vi "CIB Cal UI.vi"(11 "Calling VI Ref":refnum<vi>) -> ()   [LabVIEW 2013]
uses:
  Type Defs/Cal Point Type Def.ctl
  <vilib>/Utility/miscctls.llb/LVRowAndColumnTypeDef.ctl
panel:
  in  "debug":bool=TRUE
  in  "Load Indicator Tab":enum32{"Page 1"}(tab)
  in  "Header Tab":enum32{"Page 1", "Page 2"}(tab)
  in  "Header OK":bool
  in  "Header Cancel":bool
  in  "Header Comments":string[][](table)=[["PRODUCT 5V. IS REFERENCE ONLY."], ["1"], ["2"]]
  in  "Cal Standards Table":string[][](table)=[["FLUKE MULTIMETER", "3539"], ["FLUKE CALIBRATOR", "7955"], ["", ""], ["", ""], ["", ""]]
  in  "Sys Cal Table":string[][](table)=[["CIB BD.", "DSS 9372-1"], ["D/A BD.", "DSS 9372-2"], ["", ""], ["", ""], ["", ""]]
  in  "Header Table 1":string[][](table)=[["9372blah"], ["DELPHI"], ["TL1181E"], ["EU2C397"], ["CIB/ D/A BD."], ["5 VOLTS"], ["NEW"], ["9087"]]
  in  "Header Table 2":string[][](table)=[["39687"], ["12"], ["40052"], ["MDC"], ["24"], ["48"], ["JUM  /   DR"]]
  in  "Main Tab":enum32{"Page 1", "Page 2"}(tab)
  in  "Address":string
  in  "Send 485 Cmd":bool
  in  "485 Command":string(combo)="p_on"
  in  "View Spreadsheet":bool
  in  "Confirm Point":bool
  in  "Header":bool
  in  "Cal Point":T1
  out "CIB SN":string caption="CIB Serial Number"
  out "Dev Table 1":string[][](table)
  in  "Actual Table 1":string[][](table)=[[""], [""], [""], [""], [""], [""], [""], [""], [""]]
  out "Actual Table 2":string[][](table)
  out "Dev Table 2":string[][](table)
  in  "Read CIB":bool
  # "System Calibration Components"
  # "Calibration Standards Used"
  # "1) Enter Header Information"
  # "Send 485 Command"
  # "2) Select Cal Point"
  # "3) Collect Data"
  # "4)  Confirm/Review"
  # "*Excel must be closed to return control to this app."
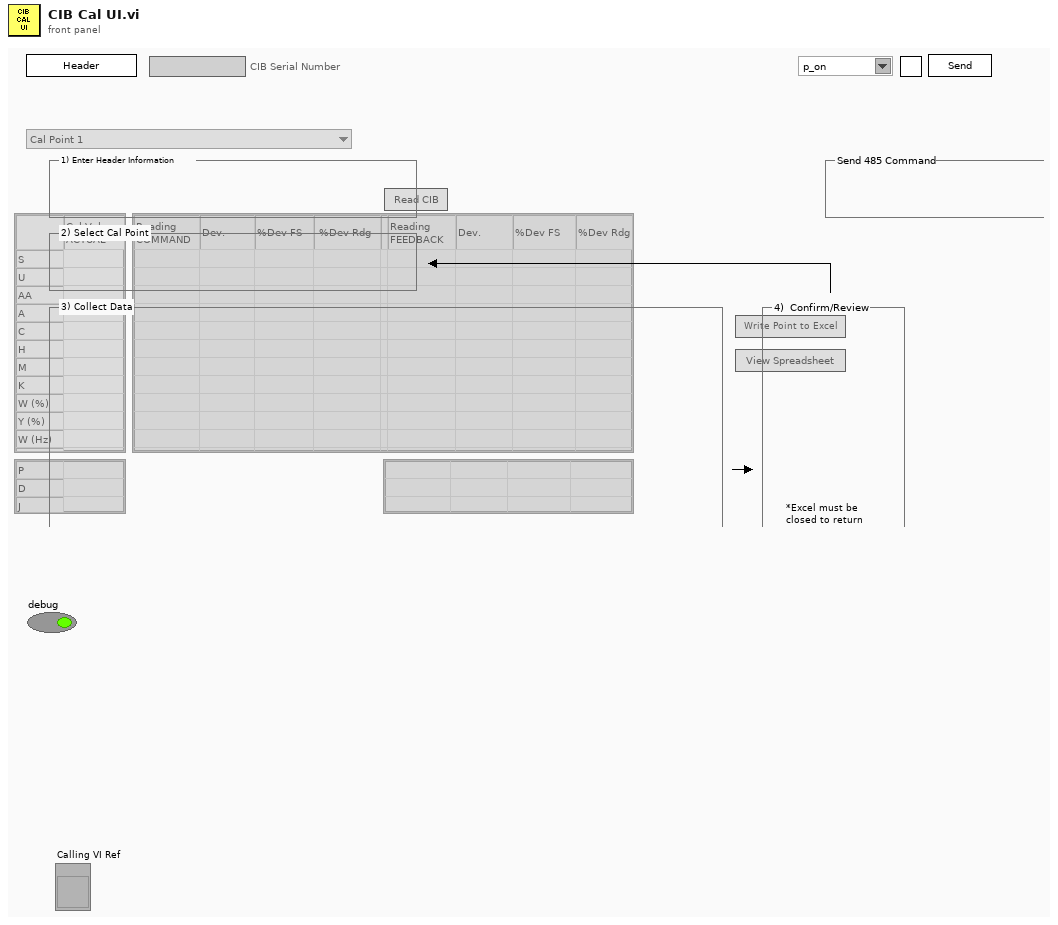
[diagram p1: front panel]
types:
  T1 = typedef "Cal Point Type Def.ctl" = enum16{"Cal Point 1", "Cal Point 2", "Cal Point 3", "Cal Point 4", "Cal Point 5", "Cal Point 6", "Cal Point 7"}
  T2 = cluster{"Error":errorcluster, "Cal Files Path":path, "Base Path":path, "Calling VI Ref":refnum<vi>, "Cal Template Path":path, "Current Cal Path":path, "Cal Point":T1, "Actual Table 1":string[][], "Actual Table 2":string[][], "Dev Table 1":string[][], "Dev Table 2":string[][], "Dev Table 1 Ref":refnum<vi>, "Dev Table 2 Ref":refnum<vi>, "COM Ref":refnum<visa-resource-name>, "COM Found":bool, "debug":bool, "Read CIB":bool}
  T3 = enum8{"Enabled", "Disabled", "Disabled and Grayed Out"}
  T4 = typedef "LVRowAndColumnTypeDef.ctl" = cluster{"Row":i32, "Column":i32}
  T5 = enum32{"Bad", "Idle", "Run top level", "Running"}
  T6 = typedef "eventvkey.ctl" = enum16{"ASCII", "Enter", "Return", "Shift", "Ctrl", "Alt", "Cmd", "Opt", "Caps", "NumLock", "Clear", "Break", "Up", "Down", "Left", "Right", "Insert", "Delete", "Home", "End", "PageUp", "PageDown", "Escape", "Help", "Pause", "ScrollLock", "F1", "F2", "F3", "F4", "F5", "F6", "F7", "F8", "F9", "F10", "F11", "F12", "F13", "F14", "F15", "F16", "F17", "F18", "F19", "F20", "F21", "F22", "F23", "F24", "Play", "VolumeUp", "VolumeDown", "Mute", "Two Byte Char"}
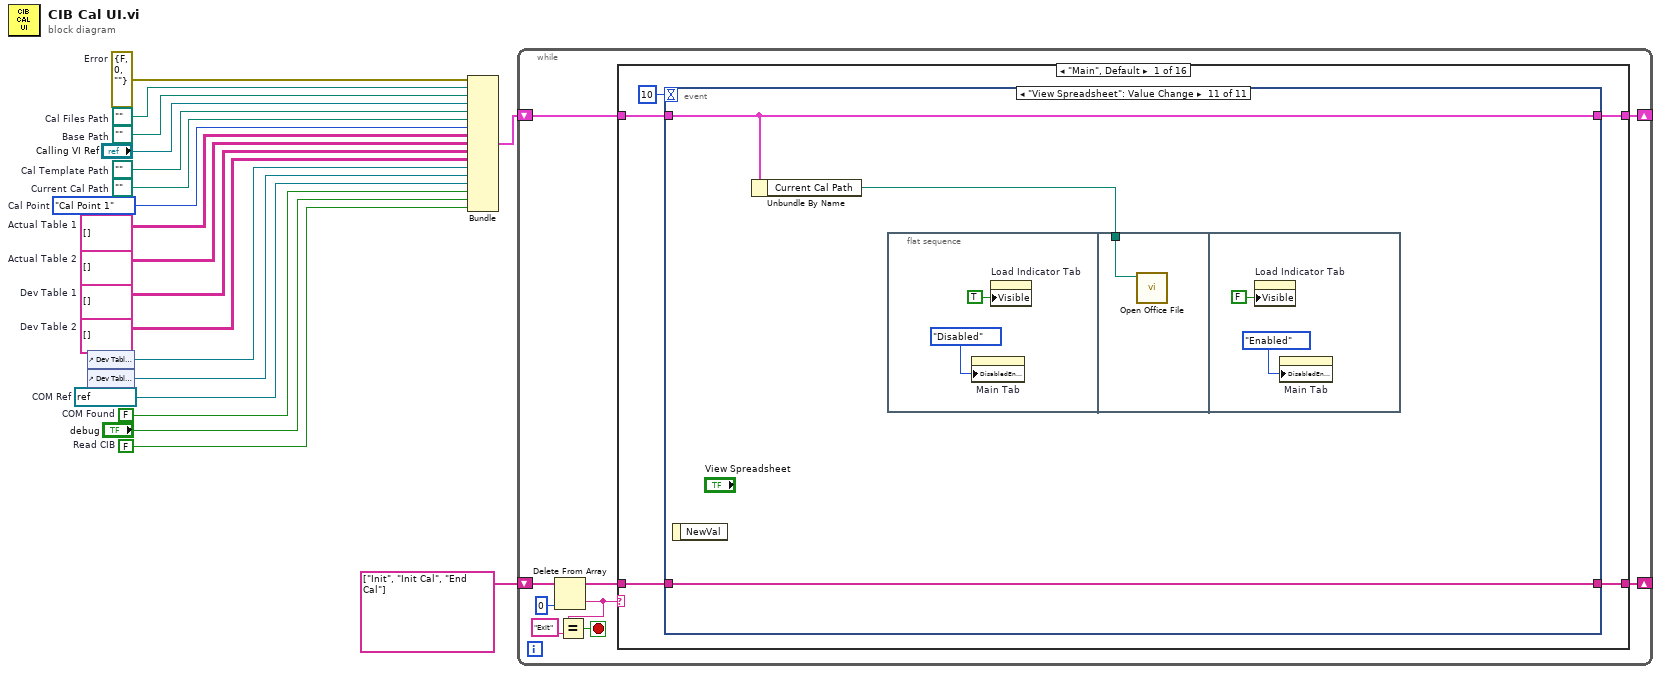
[diagram p0: block diagram]
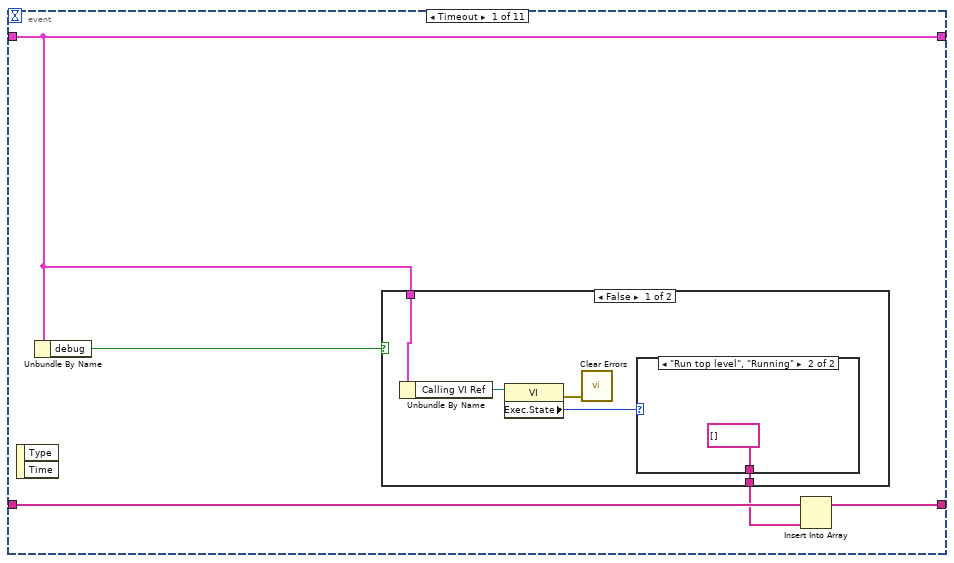
[diagram p2: hidden frame]
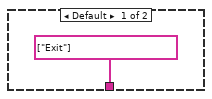
[diagram p3: hidden frame]
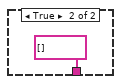
[diagram p4: hidden frame]
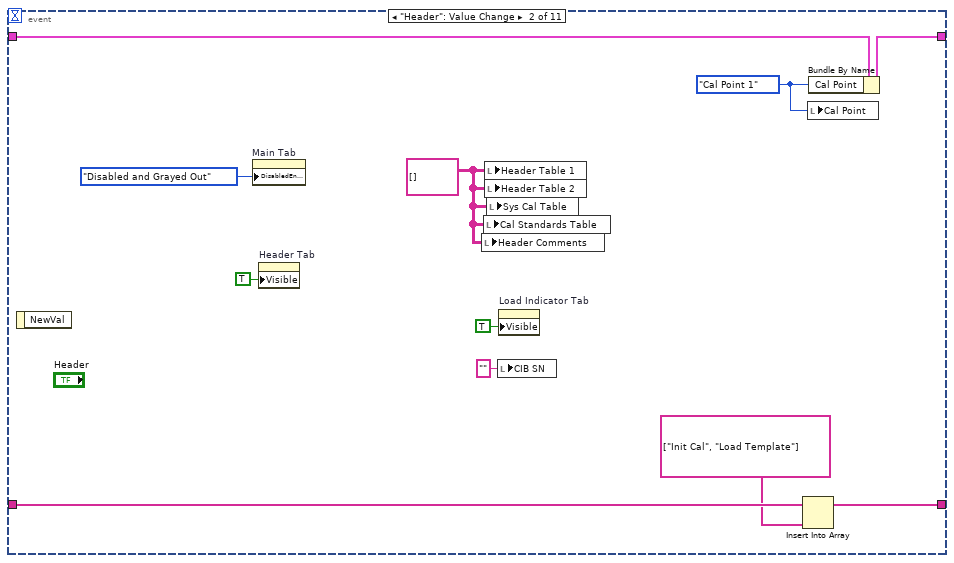
[diagram p5: hidden frame]
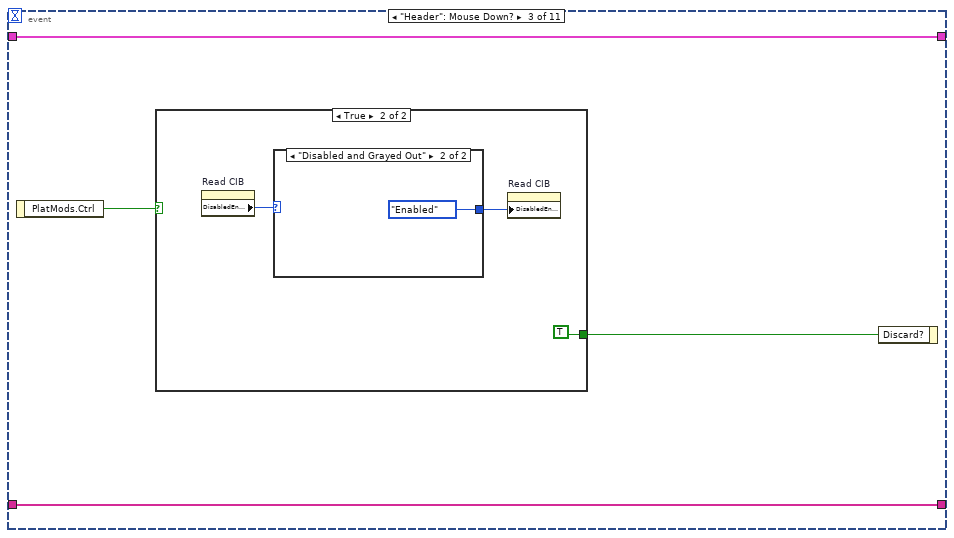
[diagram p6: hidden frame]
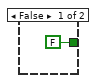
[diagram p7: hidden frame]
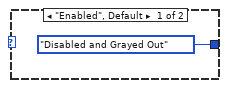
[diagram p8: hidden frame]
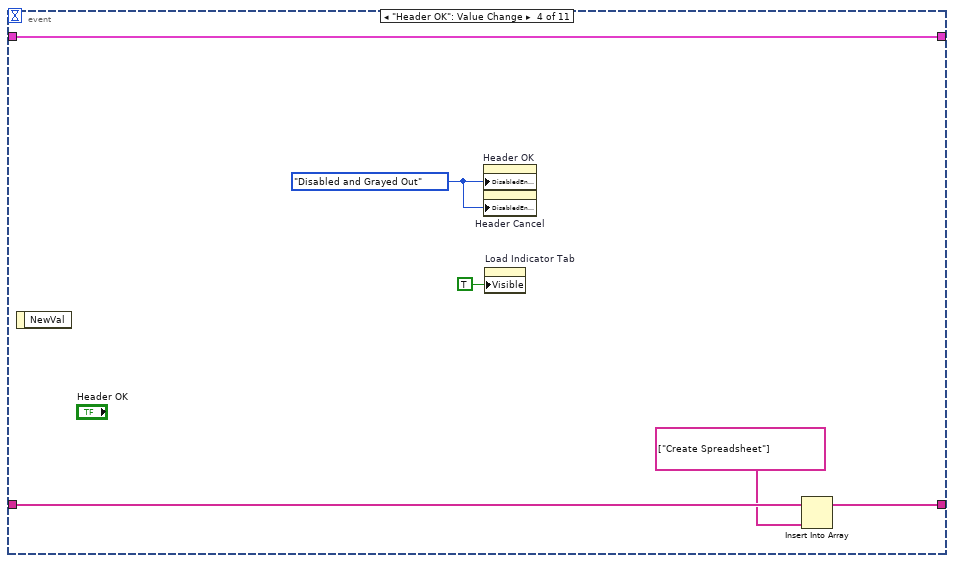
[diagram p9: hidden frame]
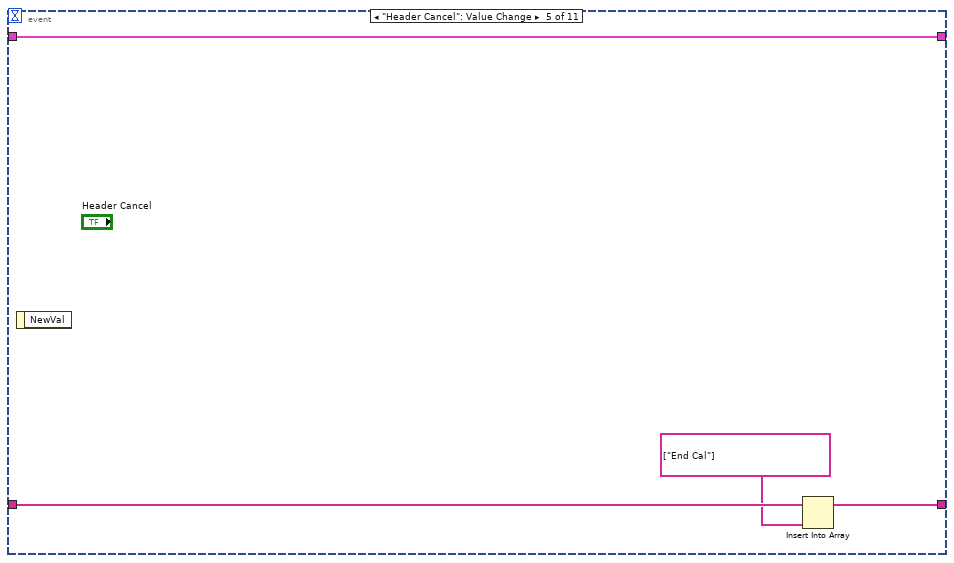
[diagram p10: hidden frame]
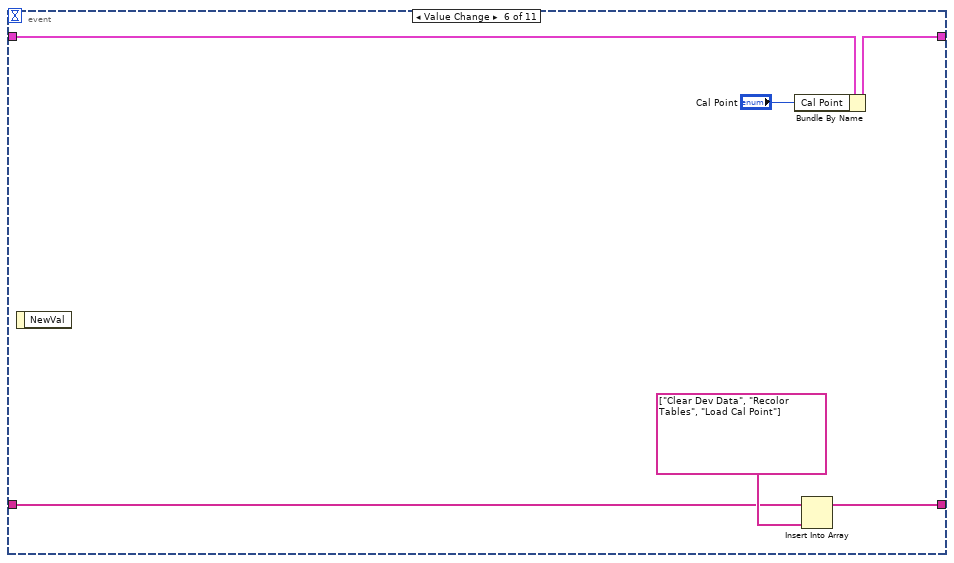
[diagram p11: hidden frame]
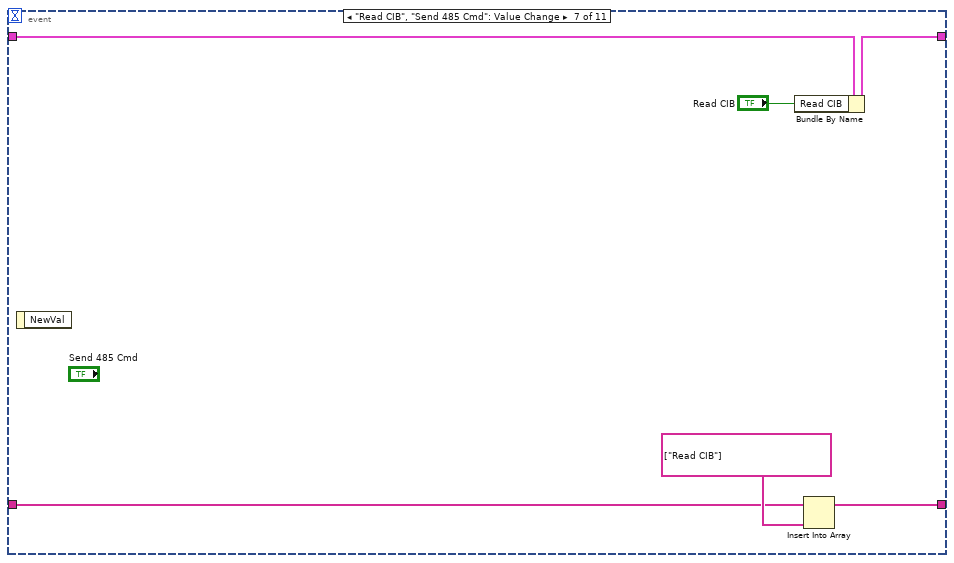
[diagram p12: hidden frame]
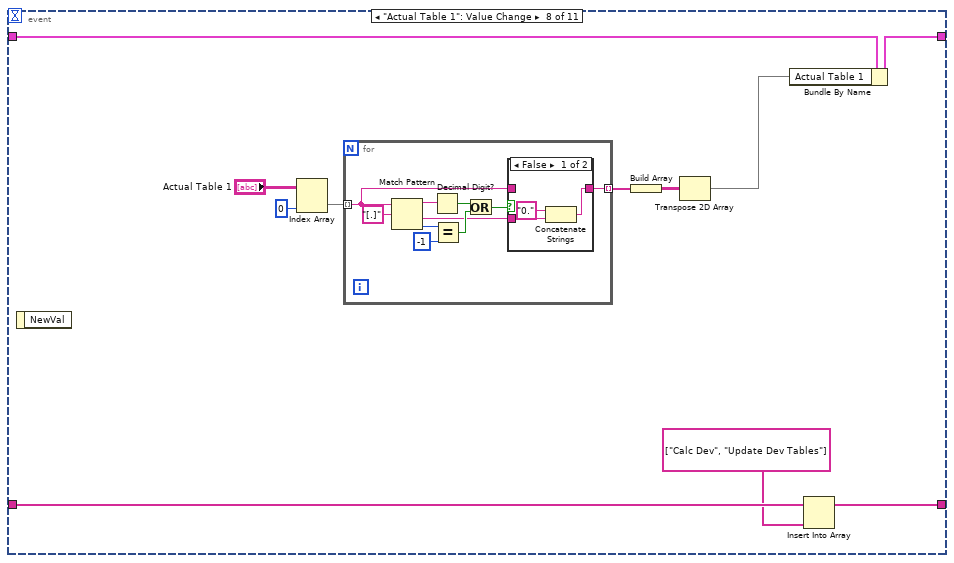
[diagram p13: hidden frame]
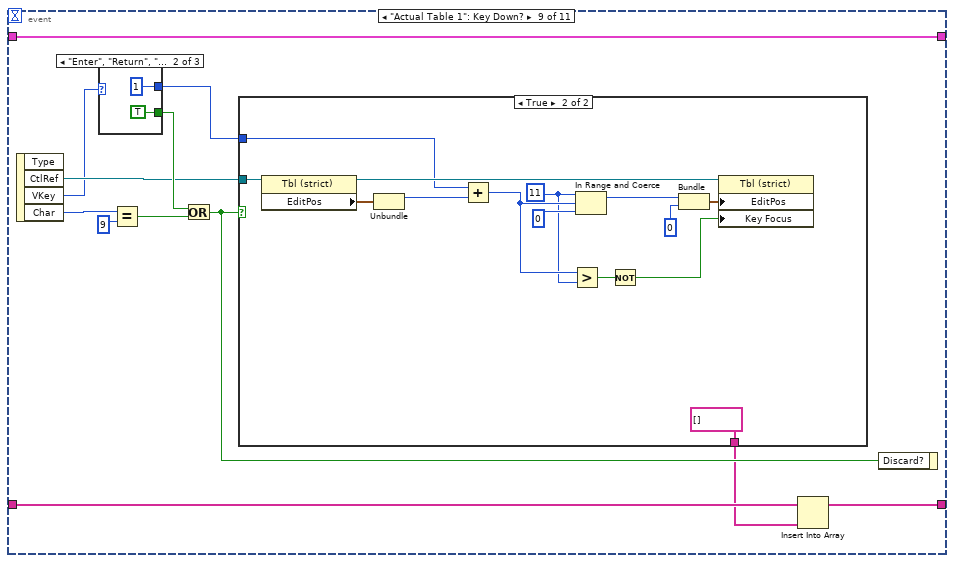
[diagram p15: hidden frame]
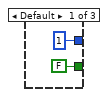
[diagram p16: hidden frame]
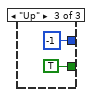
[diagram p17: hidden frame]
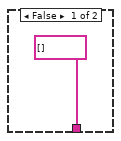
[diagram p18: hidden frame]
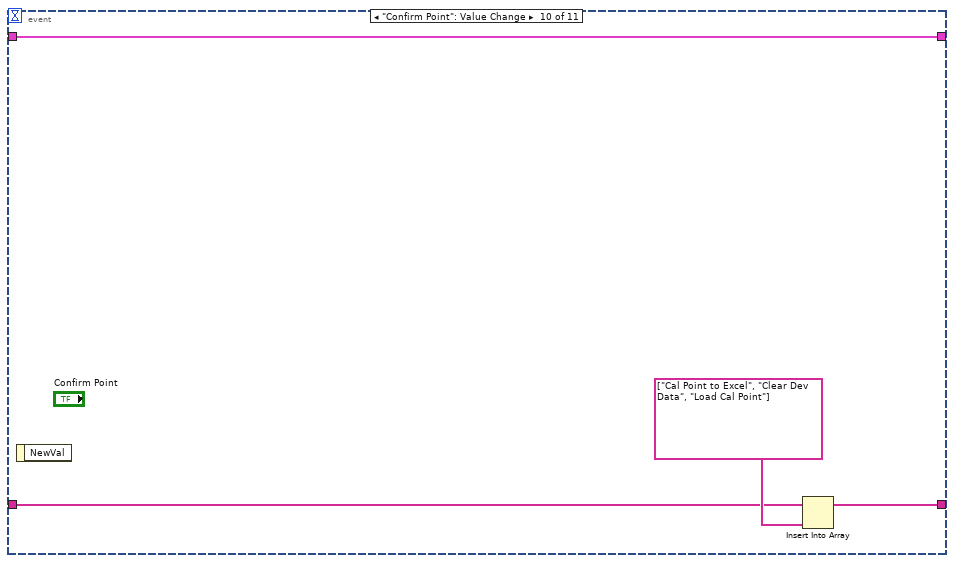
[diagram p19: hidden frame]
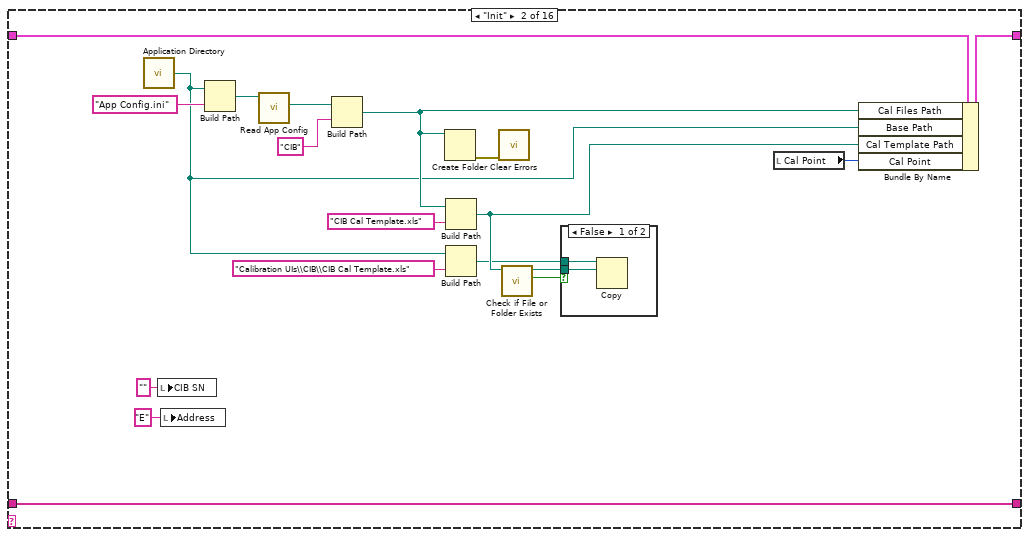
[diagram p20: hidden frame]
diagram:
  w1 = FALSE  # Read CIB
  w3 = FALSE  # COM Found
  w4 = refnum<visa-resource-name> "COM4"  # COM Ref
  w7 = string[][] []  # Dev Table 2
  w8 = string[][] []  # Dev Table 1
  w9 = string[][] []  # Actual Table 2
  w10 = string[][] []  # Actual Table 1
  w11 = Cal_Point_Type_Def."Cal Point 1"  # Cal Point
  w12 = path ""  # Current Cal Path
  w13 = path ""  # Cal Template Path
  w15 = path ""  # Base Path
  w17 = path ""  # Cal Files Path
  w16 = errorcluster {"status"=FALSE, "code"=0, "source"=""}  # Error
  n1 = control-ref of="Dev Table 1 Ref"() -> (w6:refnum<vi>)
  n2 = control-ref of="Dev Table 2 Ref"() -> (w5:refnum<vi>)
  n3 = Bundle("Error"=w16, "Cal Files Path"=w17, "Base Path"=w15, "Calling VI Ref"="Calling VI Ref", "Cal Template Path"=w13, "Current Cal Path"=w12, "Cal Point"=w11, "Actual Table 1"=w10, "Actual Table 2"=w9, "Dev Table 1"=w8, "Dev Table 2"=w7, "Dev Table 1 Ref"=w6, "Dev Table 2 Ref"=w5, "COM Ref"=w4, "COM Found"=w3, "debug"="debug", "Read CIB"=w1) -> (w18:T2)  [unwired: 1 in]
  n4 = while {
    shift-right: [w25] -> _
    shift-left: string[] ["Init", "Init Cal", "End Cal"] -> [w28]
    shift-right: [w21] -> _
    shift-left: w18 -> [w22]
    stop <- w27 stop-if-true
    n5 = Delete From Array(array=w28, index=0) -> (deleted portion=w24:string, array with subset deleted=w26:string[])  [unwired: 1 in]
    n6 = Equal?(x=w24, y="Exit" ("x")) -> (x = y?=w27:bool)
    n7 = case shown="\"Main\", Default" w24 {
      tunnel: [w31 w174 w181 w185 w194 w204 w238 w273 w309 w343 w363 w426 w455 w489 w502 w504] -> w25
      tunnel: w26 -> [w32 w174 w181 w184 w193 w203 w237 w272 w308 w342 w362 w425 w454 w489 w501 w504]
      tunnel: w22 -> [w30 w178 w182 w183 w192 w201 w229 w270 w307 w341 w366 w429 w450 w488 w493 w503]
      tunnel: [w29 w177 w182 w183 w191 w201 w228 w270 w306 w341 w365 w428 w449 w488 w493 w503] -> w21
      frame "Main", Default {
        n8 = event shown="[10] \"View Spreadsheet\": Value Change" {
          selector: _ -> [_ _ _ _ _ _ _ _ _ _ _]
          dyn-events: _ -> [_ _ _ _ _ _ _ _ _ _ _]
          timeout: 10 -> [_ _ _ _ _ _ _ _ _ _ _]
          tunnel: [w38 w57 w60 w72 w76 w79 w88 w100 w118 w150 w154] -> w31
          tunnel: w32 -> [w37 w56 w60 w71 w75 w78 w87 w99 w117 w149 w154]
          tunnel: [w35 w48 w61 w73 w77 w82 w85 w97 w115 w148 w153] -> w29
          tunnel: w30 -> [w35 w49 w61 w73 w77 w83 w86 w98 w115 w148 w153]
          event Timeout {
            n9 = event-data() -> ()  [unwired: 1 in, 2 out]
            n10 = Unbundle By Name(w35) -> ("debug"=w34:bool)
            n11 = case shown="False" w34 {
              tunnel: [w43 string[] []] -> w36
              tunnel: w35 -> [w40 _]
              frame False {
                n12 = Unbundle By Name(w40) -> ("Calling VI Ref"=w42:refnum<vi>)
                n13 = property class="VI"(reference=w42) -> (error out=w39:errorcluster, "Exec.State"=w41:T5)  [unwired: 1 in, 1 out]
                n14 = call <vilib>:"Clear Errors.vi"("error in (no error)"=w39) -> ()  [unwired: 6 in, 1 out]
                n15 = case shown="\"Run top level\", \"Running\"" w41 {
                  tunnel: [string[] ["Exit"] string[] []] -> w43
                  frame Default {
                  }
                  frame "Run top level", "Running" {
                  }
                }
              }
              frame True {
              }
            }
            n16 = Insert Into Array(array=w37, new element=w36) -> (w38:string[])  [unwired: 1 in]
          }
          event "Header": Value Change {
            w47 = Cal_Point_Type_Def."Cal Point 1" ("Cal Point")
            w53 = string[][] [] ("Header Table 1")
            n17 = event-data() -> ()  [unwired: 1 in, 1 out]
            n18 = property on="Main Tab" class="TabCtl (strict)"("DisabledEnum"=T3."Disabled and Grayed Out" ("Disabled")) -> ()  [unwired: 2 in, 2 out]
            n19 = property on="Header Tab" class="TabCtl (strict)"("Visible"=TRUE) -> ()  [unwired: 2 in, 2 out]
            n20 = local write "Header Comments"(w53) -> ()
            n21 = local write "Cal Standards Table"(w53) -> ()
            n22 = local write "Header Table 1"(w53) -> ()
            n23 = local write "Header Table 2"(w53) -> ()
            n24 = local write "Sys Cal Table"(w53) -> ()
            n25 = local write "CIB SN"("" ("CIB SN")) -> ()
            n26 = property on="Load Indicator Tab" class="TabCtl (strict)"("Visible"=TRUE) -> ()  [unwired: 2 in, 2 out]
            n27 = Insert Into Array(array=w56, new element=string[] ["Init Cal", "Load Template"]) -> (w57:string[])  [unwired: 1 in]
            n28 = local write "Cal Point"(w47) -> ()
            n29 = Bundle By Name(cluster=w49, "Cal Point"=w47) -> (w48:T2)
          }
          event "Header": Mouse Down? {
            n30 = event-data() -> ("PlatMods.Ctrl"=w59:bool)  [unwired: 1 in]
            n31 = case shown="True" w59 {
              tunnel: [FALSE TRUE] -> w58
              frame False {
              }
              frame True {
                n32 = property on="Read CIB" class="Bool"() -> ("DisabledEnum"=w65:T3)  [unwired: 2 in, 2 out]
                n33 = case shown="\"Disabled and Grayed Out\"" w65 {
                  tunnel: [T3."Disabled and Grayed Out" ("Disabled") T3."Enabled" ("Disabled")] -> w64
                  frame "Enabled", Default {
                  }
                  frame "Disabled and Grayed Out" {
                  }
                }
                n34 = property on="Read CIB" class="Bool"("DisabledEnum"=w64) -> ()  [unwired: 2 in, 2 out]
              }
            }
            n35 = event-data("Discard?"=w58) -> ()  [unwired: 1 in, 1 out]
          }
          event "Header OK": Value Change {
            w69 = T3."Disabled and Grayed Out" ("Disabled")
            n36 = event-data() -> ()  [unwired: 1 in, 1 out]
            n37 = property on="Header OK" class="Bool"("DisabledEnum"=w69) -> ()  [unwired: 2 in, 2 out]
            n38 = property on="Header Cancel" class="Bool"("DisabledEnum"=w69) -> ()  [unwired: 2 in, 2 out]
            n39 = property on="Load Indicator Tab" class="TabCtl (strict)"("Visible"=TRUE) -> ()  [unwired: 2 in, 2 out]
            n40 = Insert Into Array(array=w71, new element=string[] ["Create Spreadsheet"]) -> (w72:string[])  [unwired: 1 in]
          }
          event "Header Cancel": Value Change {
            n41 = event-data() -> ()  [unwired: 1 in, 1 out]
            n42 = Insert Into Array(array=w75, new element=string[] ["End Cal"]) -> (w76:string[])  [unwired: 1 in]
          }
          event Value Change {
            n43 = event-data() -> ()  [unwired: 1 in, 1 out]
            n44 = Bundle By Name(cluster=w83, "Cal Point"="Cal Point") -> (w82:T2)
            n45 = Insert Into Array(array=w78, new element=string[] ["Clear Dev Data", "Recolor Tables", "Load Cal Point"]) -> (w79:string[])  [unwired: 1 in]
          }
          event "Read CIB", "Send 485 Cmd": Value Change {
            n46 = event-data() -> ()  [unwired: 1 in, 1 out]
            n47 = Bundle By Name(cluster=w86, "Read CIB"="Read CIB") -> (w85:T2)
            n48 = Insert Into Array(array=w87, new element=string[] ["Read CIB"]) -> (w88:string[])  [unwired: 1 in]
          }
          event "Actual Table 1": Value Change {
            n49 = event-data() -> ()  [unwired: 1 in, 1 out]
            n50 = Index Array(array="Actual Table 1", index (col)=0 ("disabled index (col)")) -> (element=w94:string[])  [unwired: 1 in]
            n51 = for {
              tunnel: w94 -> [w103] mode=indexing
              tunnel: [w101] -> w93 mode=indexing
              n52 = Match Pattern(string=w103, regular expression="[.]") -> (before substring=w109:string, after substring=w102:string, offset past match=w107:i32)  [unwired: 1 in, 1 out]
              n53 = Decimal Digit?(1:w109) -> (0:w108:bool)
              n54 = Equal?(x=w107, y=-1) -> (x = y?=w105:bool)
              n55 = Or(x=w108, y=w105) -> (x .or. y?=w104:bool)
              n56 = case shown="False" w104 {
                tunnel: [w111 w114] -> w101
                tunnel: w103 -> [_ w114]
                tunnel: w102 -> [w113 _]
                frame False {
                  n57 = Concatenate Strings("0." ("string"), w113) -> (w111:string)
                }
                frame True {
                }
              }
            }
            n58 = Build Array(w93) -> (w92:string[][])
            n59 = Transpose 2D Array(2D array=w92) -> (transposed array=w90:string[][])
            n60 = Bundle By Name(cluster=w98, "Actual Table 1"=w90) -> (w97:T2)
            n61 = Insert Into Array(array=w99, new element=string[] ["Calc Dev", "Update Dev Tables"]) -> (w100:string[])  [unwired: 1 in]
          }
          event "Actual Table 1": Key Down? {
            n62 = event-data() -> ("CtlRef"=w122:refnum<vi>, "VKey"=w120:T6, "Char"=w121:i16)  [unwired: 1 in, 1 out]
            n63 = case shown="\"Enter\", \"Return\", \"Down\"" w120 {
              tunnel: [1 ("Column") 1 ("Column") -1 ("Column")] -> w125
              tunnel: [FALSE TRUE TRUE] -> w126
              frame Default {
              }
              frame "Enter", "Return", "Down" {
              }
              frame "Up" {
              }
            }
            n64 = Equal?(x=w121, y=i16 9) -> (x = y?=w123:bool)
            n65 = Or(x=w126, y=w123) -> (x .or. y?=w119:bool)
            n66 = case shown="True" w119 {
              tunnel: w122 -> [_ w147]
              tunnel: w125 -> [_ w142]
              tunnel: [string[] [] string[] []] -> w116
              frame False {
              }
              frame True {
                w136 = 11 ("y")
                n67 = property class="Tbl (strict)"(reference=w147) -> (reference out=w144:refnum<vi>, "EditPos"=w146:T4)  [unwired: 1 in, 1 out]
                n68 = Unbundle(w146) -> ("Row"=w141:i32)  [unwired: 1 out]
                n69 = Add(x=w142, y=w141) -> (x+y=w137:i32)
                n70 = Greater?(x=w137, y=w136) -> (0:w135:bool)
                n71 = In Range and Coerce(upper limit=w136, x=w137, lower limit=0) -> (coerced(x)=w140:i32)  [unwired: 1 out]
                n72 = Not(x=w135) -> (.not. x?=w134:bool)
                n73 = Bundle("y"=w140, "Column"=0) -> (w145:cluster{"y":i32, "Column":i32})  [unwired: 1 in]
                n74 = property class="Tbl (strict)"(reference=w144, "EditPos"=w145, "Key Focus"=w134) -> ()  [unwired: 1 in, 2 out]
              }
            }
            n75 = Insert Into Array(array=w117, new element=w116) -> (w118:string[])  [unwired: 1 in]
            n76 = event-data("Discard?"=w119) -> ()  [unwired: 1 in, 1 out]
          }
          event "Confirm Point": Value Change {
            n77 = event-data() -> ()  [unwired: 1 in, 1 out]
            n78 = Insert Into Array(array=w149, new element=string[] ["Cal Point to Excel", "Clear Dev Data", "Load Cal Point"]) -> (w150:string[])  [unwired: 1 in]
          }
          event "View Spreadsheet": Value Change {
            n79 = event-data() -> ()  [unwired: 1 in, 1 out]
            n80 = Unbundle By Name(w153) -> ("Current Cal Path"=w152:path)
            n81 = flat-sequence {
              tunnel: w152 -> [w157]
              frame #0 {
                n82 = property on="Main Tab" class="TabCtl (strict)"("DisabledEnum"=T3."Disabled" ("Disabled")) -> ()  [unwired: 2 in, 2 out]
                n83 = property on="Load Indicator Tab" class="TabCtl (strict)"("Visible"=TRUE) -> ()  [unwired: 2 in, 2 out]
              }
              frame #1 {
                n84 = call "Open Office File.vi"("Selection a Word (.doc, .docx), Excel (.xls, .xlsx), or Powerpoint (.ppt, .pptx) Document..."=w157) -> ()  [unwired: 10 in, 1 out]
              }
              frame #2 {
                n85 = property on="Load Indicator Tab" class="TabCtl (strict)"("Visible"=FALSE) -> ()  [unwired: 2 in, 2 out]
                n86 = property on="Main Tab" class="TabCtl (strict)"("DisabledEnum"=T3."Enabled" ("Disabled")) -> ()  [unwired: 2 in, 2 out]
              }
            }
          }
        }
      }
      frame "Init" {
        n87 = call <vilib>:"Application Directory.vi"() -> ("Application Directory"=w161:path)
        n88 = local write "CIB SN"("" ("CIB SN")) -> ()
        n89 = local write "Address"("E" ("Address")) -> ()
        n90 = Build Path(base path=w161, name or relative path="App Config.ini") -> (appended path=w171:path)
        n91 = call "Read App Config.vi"("App Config Path"=w171) -> ("Cal Files Path"=w173:path)  [unwired: 9 in, 1 out]
        n92 = Build Path(base path=w173, name or relative path="CIB") -> (appended path=w169:path)
        n93 = Create Folder(path (use dialog)=w169) -> (error out=w175:errorcluster)  [unwired: 2 in, 2 out]
        n94 = Build Path(base path=w169, name or relative path="CIB Cal Template.xls") -> (appended path=w166:path)
        n95 = Build Path(base path=w161, name or relative path="Calibration UIs\\CIB\\CIB Cal Template.xls") -> (appended path=w162:path)
        n96 = call <vilib>:"Clear Errors.vi"("error in (no error)"=w175) -> ()  [unwired: 6 in, 1 out]
        n97 = call <vilib>:"Check if File or Folder Exists.vi"("path"=w166) -> ("file or folder exists?"=w165:bool, "dup path"=w164:path)  [unwired: 8 in, 1 out]
        n98 = case shown="False" w165 {
          tunnel: w164 -> [w180 _]
          tunnel: w162 -> [w179 _]
          frame False {
            n99 = Copy(10:w180, 11:w179) -> ()  [unwired: 3 in, 3 out]
          }
          frame True {
          }
        }
        n100 = local read "Cal Point"() -> (w168:T1)
        n101 = Bundle By Name(cluster=w178, "Cal Files Path"=w169, "Base Path"=w161, "Cal Template Path"=w166, "Cal Point"=w168) -> (w177:T2)
      }
      frame "Unused Items" {
      }
      frame "Init Cal" {
        n102 = Insert Into Array(array=w184, new element=string[] ["Clear Dev Data", "Update Dev Tables"]) -> (w185:string[])  [unwired: 1 in]
      }
      frame "Clear Dev Data" {
        w187 = string[][] [["", "", "", ""], ["", "", "", ""], ["", "", "", ""]]  # Dev Table 2
        w188 = string[][] [["", "", "", "", "", "", "", "", ""], ["", "", "", "", "", "", "", "", ""], ["", "", "", "", "", "", "", "", ""], ["", "", "", "", "", "", "", "", ""], ["", "", "", "", "", "", "", "", ""], ["", "", "", "", "", "", "", "", ""], ["", "", "", "", "", "", "", "", ""], ["", "", "", "", "", "", "", "", ""], ["", "", "", "", "", "", "", "", ""], ["", "", "", "", "", "", "", "", ""], ["", "", "", "", "", "", "", "", ""], ["", "", "", "", "", "", "", "", ""]]  # Dev Table 1
        w189 = string[][] [[""], [""], [""]]  # Actual Table 2
        w190 = string[][] [[""], [""], [""], [""], [""], [""], [""], [""], [""], [""], [""], [""]]  # Actual Table 1
        n103 = Bundle By Name(cluster=w192, "Actual Table 1"=w190, "Actual Table 2"=w189, "Dev Table 1"=w188, "Dev Table 2"=w187) -> (w191:T2)
        n104 = Insert Into Array(array=w193, new element=string[] []) -> (w194:string[])  [unwired: 1 in]
      }
      frame "Load Template" {
        n105 = Unbundle By Name(w201) -> ("Cal Template Path"=w199:path)
        n106 = call <vilib>:"Check if File or Folder Exists.vi"("path"=w199) -> ("file or folder exists?"=w200:bool)  [unwired: 8 in, 2 out]
        n107 = case shown="False" w200 {
          tunnel: [string[] ["End Cal"] string[] []] -> w202
          tunnel: w199 -> [w208 w219]
          tunnel: [FALSE ("Visible") FALSE ("Visible")] -> w198
          tunnel: [w205 w211] -> w197
          tunnel: [w205 w211] -> w196
          frame False {
            w205 = T3."Disabled and Grayed Out" ("Disabled")
            n108 = Format Into String(format string="Can't find cal spreadsheet template!\n\nShould have been here:  \"%s\"" ("message"), w208) -> (resulting string=w207:string)  [unwired: 2 in, 1 out]
            n109 = One Button Dialog(message=w207) -> ()  [unwired: 1 in, 1 out]
          }
          frame True {
            w211 = T3."Enabled" ("Disabled")
            n110 = call "Read Write Header.vi"("Cal Template Path"=w219, "Write (F)"=FALSE) -> ("Header Table 1"=w218:string[][], "Header Table 2"=w217:string[][], "Sys Cal Table"=w214:string[][], "Cal Standards Table"=w213:string[][], "Header Comments"=w215:string[][])  [unwired: 13 in]
            n111 = local write "Header Comments"(w215) -> ()
            n112 = local write "Cal Standards Table"(w213) -> ()
            n113 = local write "Header Table 1"(w218) -> ()
            n114 = local write "Header Table 2"(w217) -> ()
            n115 = local write "Sys Cal Table"(w214) -> ()
          }
        }
        n116 = property on="Load Indicator Tab" class="TabCtl (strict)"("Visible"=w198) -> ()  [unwired: 2 in, 2 out]
        n117 = property on="Header OK" class="Bool"("DisabledEnum"=w197) -> ()  [unwired: 2 in, 2 out]
        n118 = property on="Header Cancel" class="Bool"("DisabledEnum"=w196) -> ()  [unwired: 2 in, 2 out]
        n119 = Insert Into Array(array=w203, new element=w202) -> (w204:string[])  [unwired: 1 in]
      }
      frame "Create Spreadsheet" {
        n120 = local read "Header Table 1"() -> (w235:string[][])
        n121 = Unbundle By Name(w229) -> ("Cal Files Path"=w230:path)
        n122 = Index Array(array=w235, index (row)=3, index (col)=0 ("disabled index (col)")) -> (element=w221:string)
        n123 = Format Into String(format string="%s.xls" ("initial string"), w221) -> (resulting string=w226:string)  [unwired: 2 in, 1 out]
        n124 = Build Path(base path=w230, name or relative path=w226) -> (appended path=w225:path)
        n125 = Not A Number/Path/Refnum?(number/path/refnum=w225) -> (NaN/Path/Refnum?=w224:bool)
        n126 = Empty String/Path?(string/path=w221) -> (empty?=w223:bool)
        n127 = Build Path(base path=w230, name or relative path="CIB Cal Template.xls") -> (appended path=w227:path)
        n128 = Or(x=w224, y=w223) -> (x .or. y?=w222:bool)
        n129 = case shown="True" w222 {
          tunnel: [w243 string[] []] -> w236
          tunnel: w225 -> [w240 _]
          tunnel: w227 -> [w239 _]
          frame False {
            n130 = call <vilib>:"Check if File or Folder Exists.vi"("path"=w240) -> ("file or folder exists?"=w242:bool)  [unwired: 8 in, 2 out]
            n131 = case shown="True" w242 {
              tunnel: [FALSE ("T button?") w247] -> w241
              frame False {
              }
              frame True {
                n132 = Two Button Dialog(message="Cal file already exists.  How do you want to proceed?\n\n\"Use Existing\" will continue with existing file and data.  \"Overwrite\" will destroy all data and start with fresh template", 1:"Overwrite" ("F button name (\"Cancel\")"), 2:"Use Existing" ("T button name (\"OK\")")) -> (T button?=w247:bool)
              }
            }
            n133 = case shown="False" w241 {
              tunnel: [string[] ["Save Header"] string[] ["Save Header"]] -> w243
              tunnel: w240 -> [w251 _]
              tunnel: w239 -> [w250 _]
              frame False {
                n134 = Copy(9:TRUE ("overwrite (F)"), 10:w251, 11:w250) -> ()  [unwired: 2 in, 3 out]
              }
              frame True {
              }
            }
          }
          frame True {
            w254 = T3."Enabled" ("Disabled")
            n135 = property on="Load Indicator Tab" class="TabCtl (strict)"("Visible"=FALSE) -> ()  [unwired: 2 in, 2 out]
            n136 = property on="Header OK" class="Bool"("DisabledEnum"=w254) -> ()  [unwired: 2 in, 2 out]
            n137 = property on="Header Cancel" class="Bool"("DisabledEnum"=w254) -> ()  [unwired: 2 in, 2 out]
            n138 = One Button Dialog(message="\"Manufacturer Serial #\" is blank or contains invalid characters.") -> ()  [unwired: 1 in, 1 out]
          }
        }
        n139 = Bundle By Name(cluster=w229, "Current Cal Path"=w225) -> (w228:T2)
        n140 = Insert Into Array(array=w237, new element=w236) -> (w238:string[])  [unwired: 1 in]
      }
      frame "Save Header" {
        n141 = Unbundle By Name(w270) -> ("Current Cal Path"=w260:path, "Cal Template Path"=w259:path)
        n142 = Build Array(w260, w259) -> (w258:path[])
        n143 = Index Array(array="Header Table 1", index (row)=3, index (col)=0 ("disabled index (col)")) -> (element=→"CIB SN":string)
        n144 = for {
          tunnel: "Header Table 2" -> [w281]
          tunnel: "Sys Cal Table" -> [w280]
          tunnel: "Cal Standards Table" -> [w279]
          tunnel: "Header Comments" -> [w278]
          tunnel: [w277] -> w265
          tunnel: "Header Table 1" -> [w275]
          tunnel: w258 -> [w274] mode=indexing
          n145 = call "Read Write Header.vi"("Header Table 1 IN"=w275, "Header Table 2 IN"=w281, "Sys Cal Table IN"=w280, "Cal Standards Table IN"=w279, "Header Comments IN"=w278, "Cal Template Path"=w274, "Write (F)"=TRUE) -> ("Header Table 1"=w277:string[][])  [unwired: 8 in, 4 out]
        }
        n146 = flat-sequence {
          tunnel: w265 -> [_]
          frame #0 {
            w283 = T3."Enabled" ("Disabled")
            w282 = T3."Enabled" ("Disabled")
            w284 = FALSE ("Visible")
            n147 = property on="Load Indicator Tab" class="TabCtl (strict)"("Visible"=w284) -> ()  [unwired: 2 in, 2 out]
            n148 = property on="Header Tab" class="TabCtl (strict)"("Visible"=w284) -> ()  [unwired: 2 in, 2 out]
            n149 = property on="Main Tab" class="TabCtl (strict)"("DisabledEnum"=w282) -> ()  [unwired: 2 in, 2 out]
            n150 = property on="Confirm Point" class="Bool"("DisabledEnum"=w282) -> ()  [unwired: 2 in, 2 out]
            n151 = property on="Cal Point" class="Enum (strict)"("DisabledEnum"=w282) -> ()  [unwired: 2 in, 2 out]
            n152 = property on="CIB SN" class="Str"("DisabledEnum"=w282) -> ()  [unwired: 2 in, 2 out]
            n153 = property on="Actual Table 1" class="Tbl (strict)"("DisabledEnum"=w283) -> ()  [unwired: 2 in, 2 out]
            n154 = property on="Actual Table 2" class="Tbl (strict)"("DisabledEnum"=w283) -> ()  [unwired: 2 in, 2 out]
            n155 = property on="Dev Table 1" class="Tbl (strict)"("DisabledEnum"=w283) -> ()  [unwired: 2 in, 2 out]
            n156 = property on="Dev Table 2" class="Tbl (strict)"("DisabledEnum"=w283) -> ()  [unwired: 2 in, 2 out]
            n157 = property on="Read CIB" class="Bool"("DisabledEnum"=w283) -> ()  [unwired: 2 in, 2 out]
            n158 = property on="View Spreadsheet" class="Bool"("DisabledEnum"=w283) -> ()  [unwired: 2 in, 2 out]
          }
        }
        n159 = Insert Into Array(array=w272, new element=string[] ["Load Cal Point"]) -> (w273:string[])  [unwired: 1 in]
      }
      frame "Load Cal Point" {
        n160 = Unbundle By Name(w307) -> ("Dev Table 1"=w296:string[][], "Actual Table 2"=w292:string[][], "Cal Point"=w297:T1)
        n161 = case shown="\"Cal Point 1\", Default" w297 {
          tunnel: ["0" "0.5" "1" "2" "3" "4" "5"] -> w298
          tunnel: ["20" "40" "50" "60" "80" w332 w335] -> w302
          tunnel: ["4000" "4000" "4000" "4000" "4000" w332 w335] -> w289
          tunnel: ["0" "3" "6" "9" "12" "15" "18"] -> w285
          frame "Cal Point 1", Default {
          }
          frame "Cal Point 2" {
          }
          frame "Cal Point 3" {
          }
          frame "Cal Point 4" {
          }
          frame "Cal Point 5" {
          }
          frame "Cal Point 6" {
            w332 = "na"
          }
          frame "Cal Point 7" {
            w335 = "na"
          }
        }
        n162 = Initialize Array(w298, 8 ("dimension size")) -> (w300:string[])
        n163 = Initialize Array(w302, 2 ("dimension size")) -> (w299:string[])
        n164 = Initialize Array(w289, 2 ("dimension size")) -> (w288:string[])
        n165 = Initialize Array(w298, 2 ("dimension size")) -> (w287:string[])
        n166 = Build Array (concatenate)(w300, w299, w288) -> (w294:string[])
        n167 = Build Array (concatenate)(w287, w285) -> (w286:string[])
        n168 = Replace Array Subset(array=w296, new element=w294, index (col)=0 ("disabled index (col)")) -> (w295:string[][])  [unwired: 1 in]
        n169 = Replace Array Subset(array=w292, new element=w286, index (col)=0 ("disabled index (col)")) -> (w291:string[][])  [unwired: 1 in]
        n170 = Bundle By Name(cluster=w307, "Dev Table 1"=w295, "Actual Table 2"=w291) -> (w306:T2)
        n171 = Insert Into Array(array=w308, new element=string[] ["Update Dev Tables"]) -> (w309:string[])  [unwired: 1 in]
      }
      frame "Update Dev Tables" {
        n172 = Unbundle By Name(w341) -> ("Actual Table 1"=w340:string[][], "Actual Table 2"=→"Actual Table 2":string[][], "Dev Table 1"=→"Dev Table 1":string[][], "Dev Table 2"=→"Dev Table 2":string[][])
        n173 = local write "Actual Table 1"(w340) -> ()
        n174 = Insert Into Array(array=w342, new element=string[] []) -> (w343:string[])  [unwired: 1 in]
      }
      frame "Read CIB" {
        n175 = Unbundle By Name(w366) -> ("Read CIB"=w345:bool, "Dev Table 1"=w367:string[][], "Dev Table 2"=w360:string[][], "Cal Point"=w368:T1, "COM Ref"=w358:refnum<visa-resource-name>, "COM Found"=w357:bool)
        n176 = property on="Load Indicator Tab" class="TabCtl (strict)"("Visible"=TRUE) -> (error out=w349:errorcluster)  [unwired: 2 in, 1 out]
        n177 = property on="Main Tab" class="TabCtl (strict)"("DisabledEnum"=T3."Disabled" ("Disabled")) -> (error out=w350:errorcluster)  [unwired: 2 in, 1 out]
        n178 = case shown="False" w357 {
          selector: w357 -> [_ w415]
          tunnel: [w414 w416] -> w355
          tunnel: w358 -> [_ w416]
          tunnel: [w413 w415] -> w356
          tunnel: w350 -> [_ _]
          tunnel: w349 -> [_ _]
          frame False {
            n179 = call "Find USB-485.vi"() -> ("Com Ref"=w414:refnum<visa-resource-name>, "485 Found?"=w413:bool)  [unwired: 10 in]
          }
          frame True {
          }
        }
        n180 = case shown="True" w356 {
          tunnel: w368 -> [_ w380]
          tunnel: w367 -> [w372 w379]
          tunnel: [w372 w382] -> w364
          tunnel: [string[] [] w378] -> w361
          tunnel: w360 -> [w371 w377]
          tunnel: [w371 w381] -> w359
          tunnel: w355 -> [_ w376]
          tunnel: [errorcluster {"status"=FALSE, "code"=0, "source"=""} ("Error Out") w375] -> w347
          tunnel: w345 -> [_ w374]
          frame False {
            n181 = One Button Dialog(message="Couldn't find 485 adapter!") -> ()  [unwired: 1 in, 1 out]
          }
          frame True {
            n182 = case shown="False" w374 {
              tunnel: [w388 w397] -> w382
              tunnel: [w387 w396] -> w381
              tunnel: w380 -> [_ w395]
              tunnel: w379 -> [w388 w394]
              tunnel: w377 -> [w387 w393]
              tunnel: w376 -> [w386 w392]
              tunnel: [w385 w389] -> w375
              frame False {
                n183 = call "Send 485 Command.vi"("CIB address"="Address", "COM Ref"=w386, "Message"="485 Command") -> ("Error Out"=w385:errorcluster)  [unwired: 8 in]
              }
              frame True {
                n184 = call "Read CIB.vi"("COM Ref"=w392, "Cal Point"=w395) -> ("Error Out"=w389:errorcluster, "Dev Table 2"=w390:string[][], "Dev Table 1"=w391:string[][])  [unwired: 7 in]
                n185 = case shown="No Error" w389 {
                  tunnel: w394 -> [w407 w409]
                  tunnel: [w406 w409] -> w397
                  tunnel: w391 -> [w403 _]
                  tunnel: w393 -> [w400 w408]
                  tunnel: [w399 w408] -> w396
                  tunnel: w390 -> [w398 _]
                  frame No Error {
                    n186 = Replace Array Subset(array=w407, new element=w403, index (row)=0 ("disabled index (row)"), index (col)=5 ("disabled index (col)")) -> (w406:string[][])
                    n187 = Replace Array Subset(array=w400, new element=w398, index (row)=0 ("disabled index (row)"), index (col)=0 ("disabled index (col)")) -> (w399:string[][])
                  }
                  frame Error {
                  }
                }
              }
            }
            n188 = case shown="Error" w375 {
              tunnel: [string[] ["Calc Dev", "Update Dev Tables"] string[] []] -> w378
              frame No Error {
              }
              frame Error {
                n189 = One Button Dialog(message="Error communicating with CIB.  Make sure the com port in visaconf.ini has the following settings (replace #s):\n\nName#=\"ASRL#::INSTR\"\nDisableErrorReplacement=1\nEnabled#=1\nStatic#=0\nSystemName#=\"COM#\"\nBaudRate#=19200\nDataBits#=8\nParity#=0\nStopBits#=10\nFlowCtrl#=0\n\nThe visaconf.ini may be found at:  \"C:\\Documents and Settings\\All Users\\Application Data\\National Instruments\\NIvisa\"") -> ()  [unwired: 1 in, 1 out]
              }
            }
          }
        }
        n190 = call <vilib>:"Clear Errors.vi"("error in (no error)"=w347) -> ("error out"=w346:errorcluster)  [unwired: 6 in]
        n191 = Insert Into Array(array=w362, new element=w361) -> (w363:string[])  [unwired: 1 in]
        n192 = property on="Main Tab" class="TabCtl (strict)"(error in=w346, "DisabledEnum"=T3."Enabled" ("Disabled")) -> (error out=w348:errorcluster)  [unwired: 1 in, 1 out]
        n193 = property on="Load Indicator Tab" class="TabCtl (strict)"(error in=w348, "Visible"=FALSE) -> ()  [unwired: 1 in, 2 out]
        n194 = Bundle By Name(cluster=w366, "Dev Table 1"=w364, "Dev Table 2"=w359, "COM Ref"=w355, "COM Found"=w356) -> (w365:T2)
      }
      frame "Calc Dev" {
        n195 = Unbundle By Name(w429) -> ("Actual Table 1"=w424:string[][], "Actual Table 2"=w423:string[][], "Dev Table 1"=w422:string[][], "Dev Table 2"=w421:string[][], "Dev Table 1 Ref"=w418:refnum<vi>, "Dev Table 2 Ref"=w417:refnum<vi>)
        n196 = call "Calc Dev.vi"("Actual Table 1"=w424, "Actual Table 2"=w423, "Dev Table 1"=w422, "Dev Table 2"=w421, "Dev Table 1 Ref"=w418, "Dev Table 2 Ref"=w417) -> ("Dev Table 1 OUT"=w420:string[][], "Dev Table 2 OUT"=w419:string[][])  [unwired: 12 in]
        n197 = Bundle By Name(cluster=w429, "Dev Table 1"=w420, "Dev Table 2"=w419) -> (w428:T2)
        n198 = Insert Into Array(array=w425, new element=string[] []) -> (w426:string[])  [unwired: 1 in]
      }
      frame "Cal Point to Excel" {
        n199 = Unbundle By Name(w450) -> ("Current Cal Path"=w453:path, "Actual Table 1"=w452:string[][], "Dev Table 1"=w451:string[][], "Dev Table 2"=w433:string[][], "Cal Point"=w440:T1)
        n200 = flat-sequence {
          tunnel: w440 -> [w463]
          tunnel: w451 -> [w458]
          tunnel: w452 -> [w459]
          tunnel: w453 -> [w464]
          tunnel: [w464] -> w448
          tunnel: [w459] -> w447
          tunnel: [w458] -> w446
          tunnel: [w463] -> w445
          tunnel: w440 -> [w461]
          tunnel: [w461] -> w443
          tunnel: [w459] -> w438
          tunnel: [w458] -> w436
          tunnel: [w457] -> w434
          tunnel: w433 -> [w457]
          tunnel: w448 -> [w469]
          tunnel: w447 -> [w472]
          tunnel: w446 -> [w471]
          tunnel: w445 -> [w470]
          tunnel: [w469] -> w444
          tunnel: w443 -> [w468]
          tunnel: [w468] -> w442
          tunnel: [w467] -> w439
          tunnel: w438 -> [w467]
          tunnel: [w466] -> w437
          tunnel: w436 -> [w466]
          tunnel: [w465] -> w435
          tunnel: w434 -> [w465]
          tunnel: w444 -> [w475]
          tunnel: w442 -> [w473]
          tunnel: w439 -> [w477]
          tunnel: w437 -> [w476]
          tunnel: w435 -> [w474]
          tunnel: [w475] -> w432
          tunnel: [w474] -> w431
          tunnel: [w473] -> w430
          tunnel: w432 -> [w480]
          tunnel: w431 -> [w479]
          tunnel: w430 -> [w478]
          tunnel: [w483] -> w441
          tunnel: w440 -> [w482]
          frame #0 {
            n201 = property on="Main Tab" class="TabCtl (strict)"("DisabledEnum"=T3."Disabled" ("Disabled")) -> ()  [unwired: 2 in, 2 out]
            n202 = property on="Load Indicator Tab" class="TabCtl (strict)"("Visible"=TRUE) -> ()  [unwired: 2 in, 2 out]
          }
          frame #1 {
            n203 = call "Write Sheet2 Data.vi"("Cal Point"=w470, "Dev Table 1"=w471, "Actual Table 1"=w472, "Cal Path"=w469) -> ()  [unwired: 8 in]
          }
          frame #2 {
            n204 = call "Write Sheet3 Data.vi"("Cal Path"=w475, "Actual Table 1"=w477, "Dev Table 1"=w476, "Dev Table 2"=w474, "Cal Point"=w473) -> ()  [unwired: 11 in]
          }
          frame #3 {
            n205 = call "Write Sheet4 Data.vi"("Cal Path"=w480, "Dev Table 2"=w479, "Cal Point"=w478) -> ()  [unwired: 13 in]
          }
          frame #4 {
            n206 = Increment(x=w482) -> (x+1=w483:T1)
            n207 = property on="Main Tab" class="TabCtl (strict)"("DisabledEnum"=T3."Enabled" ("Disabled")) -> ()  [unwired: 2 in, 2 out]
            n208 = property on="Load Indicator Tab" class="TabCtl (strict)"("Visible"=FALSE) -> ()  [unwired: 2 in, 2 out]
          }
        }
        n209 = Insert Into Array(array=w454, new element=string[] ["Recolor Tables"]) -> (w455:string[])  [unwired: 1 in]
        n210 = local write "Cal Point"(w441) -> ()
        n211 = Bundle By Name(cluster=w450, "Cal Point"=w441) -> (w449:T2)
      }
      frame "Recolor Tables" {
        n212 = Unbundle By Name(w488) -> ("Dev Table 1 Ref"=w487:refnum<vi>, "Dev Table 2 Ref"=w486:refnum<vi>)
        n213 = Build Array(w487, w486) -> (w485:refnum<vi>[])
        n214 = for {
          tunnel: w485 -> [w491] mode=indexing
          n215 = property on="Property Node" class="Tbl (strict)"(reference=w491, "Active Cell"=T4 {"Row"=-2, "Column"=-2} ("Active Cell:Active Cell"), "Cell BG Color"=u32 15527148) -> ()  [unwired: 1 in, 2 out]
        }
      }
      frame "End Cal" {
        w494 = T3."Disabled and Grayed Out" ("Disabled")
        w496 = T3."Disabled and Grayed Out" ("Disabled")
        w499 = T3."Disabled and Grayed Out" ("Disabled")
        n216 = property on="CIB SN" class="Str"("DisabledEnum"=w499) -> ()  [unwired: 2 in, 2 out]
        n217 = property on="Confirm Point" class="Bool"("DisabledEnum"=w499) -> ()  [unwired: 2 in, 2 out]
        n218 = property on="Cal Point" class="Enum (strict)"("DisabledEnum"=w499) -> ()  [unwired: 2 in, 2 out]
        n219 = property on="Actual Table 1" class="Tbl (strict)"("DisabledEnum"=w494) -> ()  [unwired: 2 in, 2 out]
        n220 = property on="Actual Table 2" class="Tbl (strict)"("DisabledEnum"=w494) -> ()  [unwired: 2 in, 2 out]
        n221 = property on="Dev Table 1" class="Tbl (strict)"("DisabledEnum"=w494) -> ()  [unwired: 2 in, 2 out]
        n222 = property on="Dev Table 2" class="Tbl (strict)"("DisabledEnum"=w494) -> ()  [unwired: 2 in, 2 out]
        n223 = property on="Read CIB" class="Bool"("DisabledEnum"=w494) -> ()  [unwired: 2 in, 2 out]
        n224 = property on="View Spreadsheet" class="Bool"("DisabledEnum"=w494) -> ()  [unwired: 2 in, 2 out]
        n225 = property on="Main Tab" class="TabCtl (strict)"("DisabledEnum"=T3."Enabled" ("Disabled")) -> ()  [unwired: 2 in, 2 out]
        n226 = property on="Header Tab" class="TabCtl (strict)"("Visible"=FALSE) -> ()  [unwired: 2 in, 2 out]
        n227 = property on="Load Indicator Tab" class="TabCtl (strict)"("Visible"=FALSE) -> ()  [unwired: 2 in, 2 out]
        n228 = property on="Header OK" class="Bool"("DisabledEnum"=w496) -> ()  [unwired: 2 in, 2 out]
        n229 = property on="Header Cancel" class="Bool"("DisabledEnum"=w496) -> ()  [unwired: 2 in, 2 out]
        n230 = Insert Into Array(array=w501, new element=string[] ["Recolor Tables"]) -> (w502:string[])  [unwired: 1 in]
      }
      frame "Exit" {
      }
    }
  }
